vi "edit_test_vectors.vi"() -> ()   [LabVIEW 2019]
doc: "A VI for edit test vectors of ctl_test_vector_array type.\nFunctions:\nSave Test Vector: binary write of ctl_test_vector type Test vector control into a file\nLoad Test Vector: binary read of ctl_test_vector type from file, updating the Test vector control\nDuplicate last: appending the last item to the array"
uses:
  ctl_test_vector_array.ctl
  ctl_test_item_cluster.ctl
  ctl_stimuli_cluster.ctl
  ctl_loads_enum.ctl
  ctl_pass_limits_cluster.ctl
panel:
  in  "btn_duplicate":bool
  in  "Test vector":T1
  in  "btn_load_test_vector":bool
  in  "stop":bool
  in  "btn_save_vector":bool
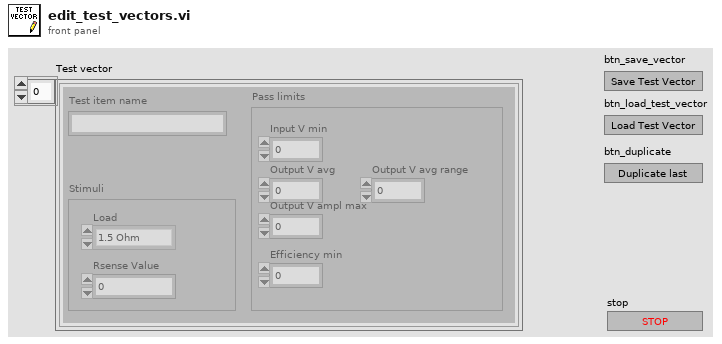
[diagram p1: front panel]
types:
  T1 = typedef "ctl_test_vector_array.ctl" = T2[]
  T2 = typedef "ctl_test_item_cluster.ctl" = cluster{"Stimuli":T3, "Pass limits":T5, "Test item name":string}
  T3 = typedef "ctl_stimuli_cluster.ctl" = cluster{"Load":T4, "Rsense Value":dbl}
  T4 = typedef "ctl_loads_enum.ctl" = enum16{"1.5 Ohm", "2.2 Ohm", "4.7 Ohm", "NO LOAD"}
  T5 = typedef "ctl_pass_limits_cluster.ctl" = cluster{"Output V avg":dbl, "Output V ampl max":dbl, "Efficiency min":dbl, "Input V min":dbl, "Output V avg range":dbl}
  T6 = enum16{"open", "replace", "create", "open or create", "replace or create", "replace or create with confirmation"}
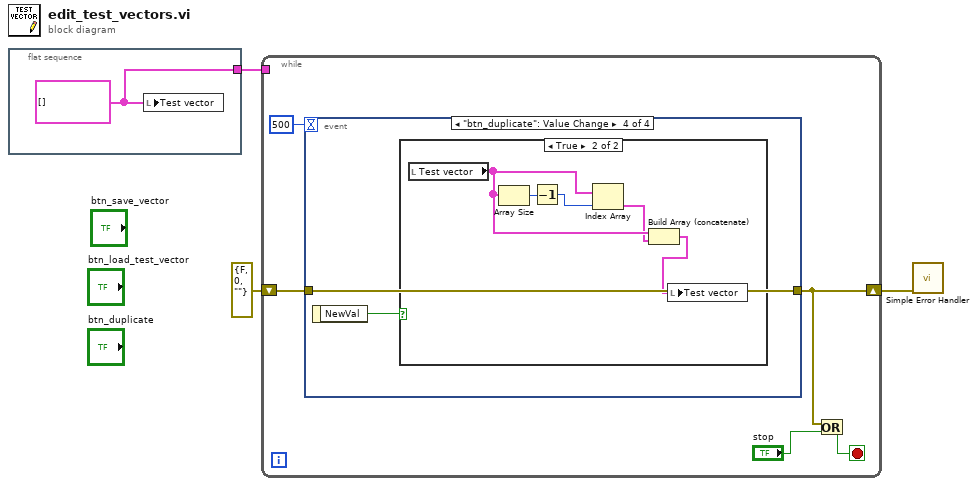
[diagram p0: block diagram]
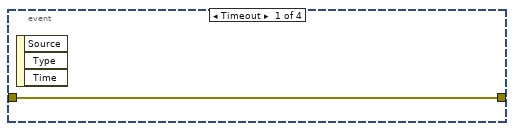
[diagram p2: hidden frame]
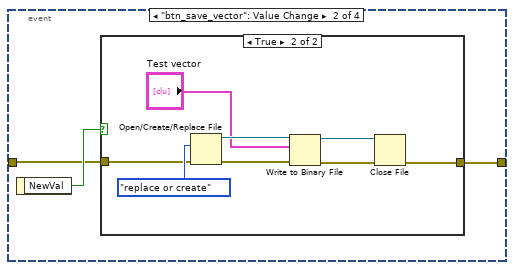
[diagram p3: hidden frame]
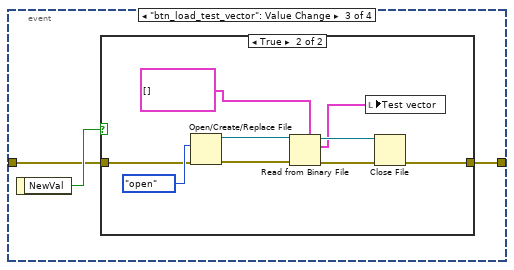
[diagram p5: hidden frame]
diagram:
  n1 = flat-sequence {
    tunnel: [w4] -> w3
    frame #0 {
      w4 = T1 [] ("Test vector")
      n2 = local write "Test vector"(w4) -> ()
    }
  }
  n3 = while {
    tunnel: w3 -> [_]
    shift-right: [w6] -> w1
    shift-left: errorcluster {"status"=FALSE, "code"=0, "source"=""} ("error out") -> [w8]
    stop <- w5 stop-if-true
    n4 = event shown="[3] \"btn_duplicate\": Value Change" {
      selector: _ -> [_ _ _ _]
      dyn-events: _ -> [_ _ _ _]
      timeout: 500 -> [_ _ _ _]
      tunnel: [w10 w12 w23 w37] -> w6
      tunnel: w8 -> [w10 w11 w24 w37]
      event Timeout {
        n5 = event-data() -> ()  [unwired: 1 in, 3 out]
      }
      event "btn_save_vector": Value Change {
        n6 = event-data() -> ("NewVal"=w13:bool)  [unwired: 1 in]
        n7 = case shown="True" w13 {
          tunnel: [w14 w17] -> w12
          tunnel: w11 -> [w14 w16]
          frame False {
          }
          frame True {
            n8 = Open/Create/Replace File(error in=w16, operation (0:open)=T6."replace or create") -> (refnum out=w22:refnum<file>, error out=w20:errorcluster)  [unwired: 4 in, 1 out]
            n9 = Write to Binary File(file (use dialog)=w22, data="Test vector", error in=w20) -> (refnum out=w21:refnum<file>, error out=w19:errorcluster)  [unwired: 3 in, 1 out]
            n10 = Close File(refnum=w21, error in=w19) -> (error out=w17:errorcluster)  [unwired: 1 out]
          }
        }
      }
      event "btn_load_test_vector": Value Change {
        n11 = event-data() -> ("NewVal"=w25:bool)  [unwired: 1 in]
        n12 = case shown="True" w25 {
          tunnel: w24 -> [w26 w30]
          tunnel: [w26 w29] -> w23
          frame False {
          }
          frame True {
            n13 = Open/Create/Replace File(error in=w30, operation (0:open)=T6."open") -> (refnum out=w35:refnum<file>, error out=w33:errorcluster)  [unwired: 4 in, 1 out]
            n14 = Read from Binary File(5:T1 [] ("Test vector"), 8:w33, 11:w35) -> (0:w32:errorcluster, 2:w28:T1, 3:w34:refnum<file>)  [unwired: 3 in, 1 out]
            n15 = local write "Test vector"(w28) -> ()
            n16 = Close File(refnum=w34, error in=w32) -> (error out=w29:errorcluster)  [unwired: 1 out]
          }
        }
      }
      event "btn_duplicate": Value Change {
        n17 = event-data() -> ("NewVal"=w36:bool)  [unwired: 1 in]
        n18 = case shown="True" w36 {
          frame False {
          }
          frame True {
            n19 = local read "Test vector"() -> (w41:T1)
            n20 = Array Size(array=w41) -> (size(s)=w42:i32)
            n21 = Decrement(x=w42) -> (x-1=w40:i32)
            n22 = Index Array(array=w41, index=w40) -> (element=w39:T2)
            n23 = Build Array (concatenate)(w41, w39) -> (w38:T1)
            n24 = local write "Test vector"(w38) -> ()
          }
        }
      }
    }
    n25 = Or(x=w6, y="stop") -> (x .or. y?=w5:bool)
  }
  n26 = call <vilib>:"Simple Error Handler.vi"("error in (no error)"=w1) -> ()  [unwired: 4 in, 5 out]
